vi "Read String Data.vi"(8 "error in (no error)":errorcluster, 11 "LV Argument Parser in":refnum<class "LV Argument Parser.lvclass">) -> (0 "error out":errorcluster, 2 "String Data":map{string, string[]}(c390), 3 "LV Argument Parser out":refnum<class "LV Argument Parser.lvclass">)   [LabVIEW 2020, in "LV ArgParse.lvlib" / "LV Argument Parser.lvclass"]
uses:
  LV Argument Parser.lvclass
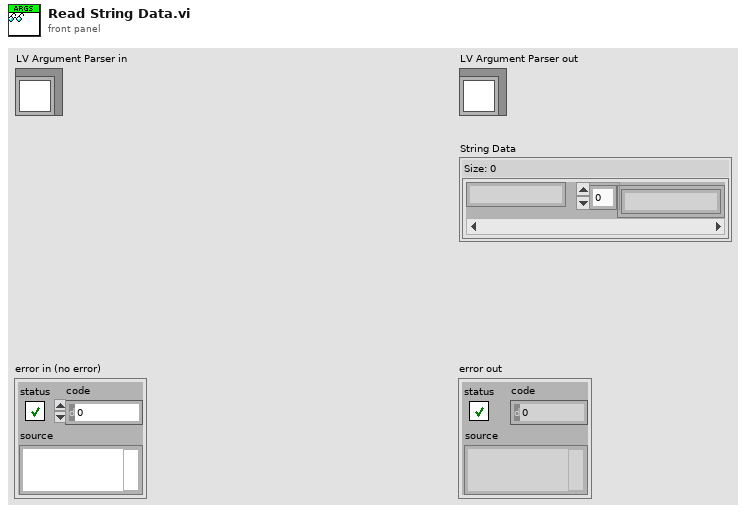
[diagram p1: front panel]
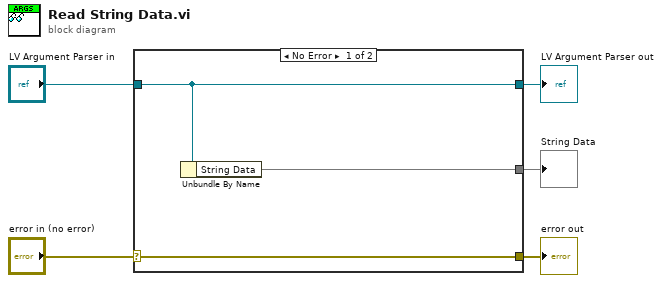
[diagram p0: block diagram]
diagram:
  n1 = case shown="No Error" "error in (no error)" {
    selector: "error in (no error)" -> [w8 w9]
    tunnel: [w8 w9] -> w4
    tunnel: [w7 w10] -> w2
    tunnel: "LV Argument Parser in" -> [w7 w10]
    tunnel: [w6 _] -> w1
    frame No Error {
      n2 = Unbundle By Name(w7) -> ("String Data"=w6:map{string, string[]})
    }
    frame Error {
    }
  }
  "error out" <- w4
  "LV Argument Parser out" <- w2
  "String Data" <- w1
